vi "CloseOpenGrip.vi"(0 "Array":bool[](array[boolean])=[TRUE, FALSE, TRUE]) -> ()   [LabVIEW 2017]
uses:
  Projekt-RubikLibrary/ServoEnumControl.ctl
  Projekt-RubikLibrary/RubikLibraryRT.lvlib
  Projekt-RubikLibrary/RubikLibrary.lvlib
panel:
  # "Close the open gripper of three!"
  # "Input:\nBoolean array of grippers states\nOnly one element is false, gripper is open.\n\nClose this gripper!"
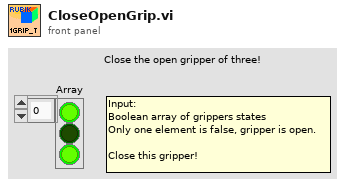
[diagram p1: front panel]
types:
  T1 = typedef "RubikLibrary.lvlib/ServoEnumControl.ctl" = enum16{"Left Servo", "Front Servo", "Right Servo"}
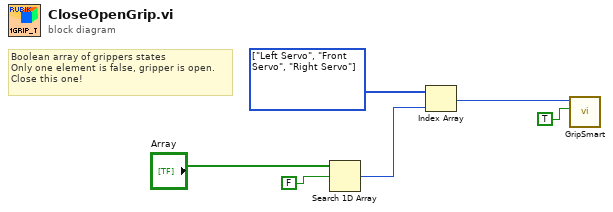
[diagram p0: block diagram]
diagram:
  w4 = T1[] [enum."Left Servo", enum."Front Servo", enum."Right Servo"] items=["Left Servo", "Front Servo", "Right Servo"]
  # "Boolean array of grippers states\nOnly one element is false, gripper is open.\nClose this one!"
  n1 = Search 1D Array(1D array="Array", element=FALSE) -> (index of element=w3:i32)  [unwired: 1 in]
  n2 = Index Array(array=w4, index=w3) -> (element=w2:T1)
  n3 = call "GripSmart.vi"("Grip closed (in)"=TRUE, "Servo"=w2) -> ()  [unwired: 8 in, 2 out]
